vi "Write mode.vi"(8 "error in (no error)":errorcluster, 10 "rqcBob Generation Mode":T1, 11 "rqcBob in":refnum<class "rqcBob.lvclass">) -> (0 "error out":errorcluster, 3 "rqcBob out":refnum<class "rqcBob.lvclass">)   [LabVIEW 2018, in "rqcBob.lvclass"]
uses:
  rqcBob.lvclass
  FPGA/rqcBob/Custom Controls/Pulse Train/rqcBob Pulse Train.Generation Mode.ctl
  Custom Controls/rqcBob Main FPGA interface.ctl
  rqcBob.lvclass/rqcBob.ctl
  <vilib>/Utility/error.llb/Error Cluster From Error Code.vi
  <vilib>/rvi/errors/niLvFpgaAdjustHostInterfaceError.vi
  <vilib>/rvi/interface/nirviReadWriteControl/nirviReadWriteControl.xnode
  NiFpgaLv.dll
  <vilib>/rvi/interface/Simulation/niFpgaSimulationCallBeginRW.vi
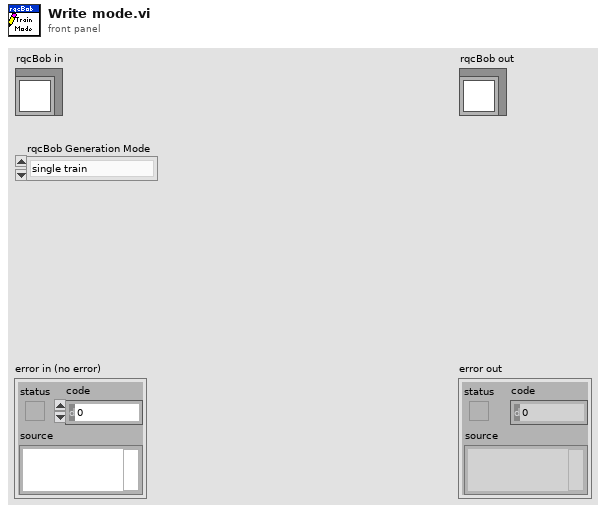
[diagram p1: front panel]
types:
  T1 = typedef "rqcBob Pulse Train.Generation Mode.ctl" = enum8{"single train", "train sequence.single", "train sequence.wait for trigger", "continuous"}
  T2 = typedef "rqcBob.lvclass/rqcBob Main FPGA interface.ctl" = refnum<k20>
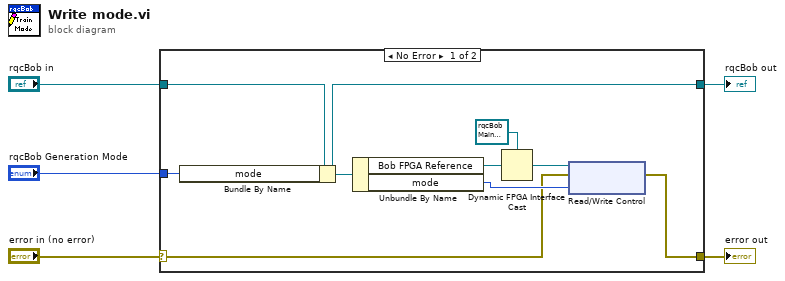
[diagram p0: block diagram]
diagram:
  n1 = case shown="No Error" "error in (no error)" {
    selector: "error in (no error)" -> [w6 w15]
    tunnel: [w7 w15] -> w4
    tunnel: [w8 w16] -> w2
    tunnel: "rqcBob in" -> [w14 w16]
    tunnel: "rqcBob Generation Mode" -> [w13 _]
    frame No Error {
      n2 = Bundle By Name(cluster=w14, "mode"=w13) -> (w8:refnum<class "rqcBob.lvclass">)
      n3 = Unbundle By Name(w8) -> ("Bob FPGA Reference"=w12:refnum<k20>, "mode"=w9:T1)
      n4 = Dynamic FPGA Interface Cast(Session In=T2 refnum ("Bob main FPGA interface"), Type=w12) -> (Session Out=w10:T2)
      n5 = xnode "Read/Write Control"("FPGA VI Reference In"=w10, "error in"=w6, "train.mode"=w9) -> ("error out"=w7:errorcluster)  [unwired: 1 out]
    }
    frame Error {
    }
  }
  "error out" <- w4
  "rqcBob out" <- w2
